vi "Main Tclk.vi"() -> ()   [LabVIEW 2018] (continued)
                n634 = call <vilib>:"Draw Rectangle.vi"("picture"=picture data[5B], "rect"=T46 {"left"=0, "top"=0, "right"=0, "bottom"=0}) -> ("new picture"=w2827:picture)  [unwired: 7 in]
                n635 = Unbundle By Name(w2823) -> ("Primary X index"=w2824:u8[][], "Primary Y index"=w2825:u8[][])
                n636 = case shown="0, Default" w2834 {
                  tunnel: w2829 -> [w2838 w2842]
                  tunnel: [w2837 w2841] -> w2828
                  tunnel: w2827 -> [w2836 w2840]
                  tunnel: [w2835 w2839] -> w2826
                  frame 0, Default {
                    n637 = Unbundle By Name(w2838) -> ("A Img Focus Index array"=w2837:dbl[][])
                    n638 = control-ref of="Detector A"() -> (w2835:refnum<vi>)
                    n639 = property on="Detector B" class="IntGraph (strict)"("PlotImages.Front"=w2836) -> ()  [unwired: 2 in, 2 out]
                  }
                  frame 1 {
                    n640 = Unbundle By Name(w2842) -> ("B Img Focus Index array"=w2841:dbl[][])
                    n641 = control-ref of="Detector B"() -> (w2839:refnum<vi>)
                    n642 = property on="Detector A" class="IntGraph (strict)"("PlotImages.Front"=w2840) -> ()  [unwired: 2 in, 2 out]
                  }
                }
                n643 = Index Array(array=w2818) -> (element #1=w2817:u8, element #2=w2816:u8)  [unwired: 2 in]
                n644 = Index Array(array=w2824, index (row)=w2817, index (col)=w2816) -> (element=w2822:u8)
                n645 = Index Array(array=w2825, index (row)=w2817, index (col)=w2816) -> (element=w2821:u8)
                n646 = call "Display array on Figure.vi"("Y resolution"=w2819, "X resolution"=w2820, "format string"="%2.3f", "Image fit to"=w2815, "Primary grid @ green"=TRUE, "Input array"=w2828, "Primary Y"=w2821, "Primary X"=w2822, "Image reference"=w2826) -> ()  [unwired: 3 in]
              }
              frame #1 {
                n647 = local read "SEM Scan Parameters"() -> (w2845:T26)
                n648 = local read "Focus Index Options"() -> (w2844:T28)
                n649 = local read "Tiled Image fit to"() -> (w2843:u8)
                n650 = call <vilib>:"Draw Rectangle.vi"("picture"=picture data[5B], "rect"=T46 {"left"=0, "top"=0, "right"=0, "bottom"=0}) -> ("new picture"=w2847:picture)  [unwired: 7 in]
                n651 = case shown="0, Default" w2850 {
                  tunnel: w2847 -> [w2852 w2854]
                  tunnel: [w2851 w2853] -> w2846
                  frame 0, Default {
                    n652 = control-ref of="Det A"() -> (w2851:refnum<vi>)
                    n653 = property on="Det B" class="IntGraph (strict)"("PlotImages.Front"=w2852) -> ()  [unwired: 2 in, 2 out]
                  }
                  frame 1 {
                    n654 = control-ref of="Det B"() -> (w2853:refnum<vi>)
                    n655 = property on="Det A" class="IntGraph (strict)"("PlotImages.Front"=w2854) -> ()  [unwired: 2 in, 2 out]
                  }
                }
                n656 = call "Display FI locations on tiled image.vi"("Tiled Image fit to"=w2843, "Focus Index Options"=w2844, "SEM Scan Parameters"=w2845, "Image reference"=w2846) -> ()  [unwired: 8 in]
              }
            }
          }
        }
        n657 = case shown="True" w2528 {
          tunnel: w2526 -> [_ w2750]
          frame False {
          }
          frame True {
            "Last good FI" <- w2750
          }
        }
        n658 = shared-variable "My Computer\\Zeiss Library.lvlib\\Image Fit to"("Image fit to") -> ()  [unwired: 1 in, 1 out]
        n659 = case shown="1" "Image fit to" {
          frame 0, Default {
            n660 = stacked-sequence {
              frame #0 {
                w2688 = u8 0 ("Y Scale.Scale Fit")
                w2689 = u8 1 ("X Scale.Scale Fit")
                n661 = property on="Detector A" class="IntGraph (strict)"("XScale.ScaleFit"=w2689) -> ()  [unwired: 2 in, 2 out]
                n662 = property on="Detector A" class="IntGraph (strict)"("YScale.ScaleFit"=w2688) -> ()  [unwired: 2 in, 2 out]
                n663 = property on="Detector B" class="IntGraph (strict)"("XScale.ScaleFit"=w2689) -> ()  [unwired: 2 in, 2 out]
                n664 = property on="Detector B" class="IntGraph (strict)"("YScale.ScaleFit"=w2688) -> ()  [unwired: 2 in, 2 out]
              }
              frame #1 {
                n665 = property on="Detector A" class="IntGraph (strict)"() -> ("XScale.Maximum"=w2691:dbl)  [unwired: 2 in, 2 out]
                n666 = property on="Detector B" class="IntGraph (strict)"() -> ("XScale.Maximum"=w2690:dbl)  [unwired: 2 in, 2 out]
                n667 = property on="Detector A" class="IntGraph (strict)"("YScale.Maximum"=w2691) -> ()  [unwired: 2 in, 2 out]
                n668 = property on="Detector B" class="IntGraph (strict)"("YScale.Maximum"=w2690) -> ()  [unwired: 2 in, 2 out]
              }
            }
          }
          frame 1 {
            n669 = stacked-sequence {
              frame #0 {
                w2692 = u8 1 ("Y Scale.Scale Fit")
                w2693 = u8 0 ("X Scale.Scale Fit")
                n670 = property on="Detector A" class="IntGraph (strict)"("XScale.ScaleFit"=w2693) -> ()  [unwired: 2 in, 2 out]
                n671 = property on="Detector A" class="IntGraph (strict)"("YScale.ScaleFit"=w2692) -> ()  [unwired: 2 in, 2 out]
                n672 = property on="Detector B" class="IntGraph (strict)"("XScale.ScaleFit"=w2693) -> ()  [unwired: 2 in, 2 out]
                n673 = property on="Detector B" class="IntGraph (strict)"("YScale.ScaleFit"=w2692) -> ()  [unwired: 2 in, 2 out]
              }
              frame #1 {
                n674 = property on="Detector A" class="IntGraph (strict)"() -> ("YScale.Maximum"=w2695:dbl)  [unwired: 2 in, 2 out]
                n675 = property on="Detector B" class="IntGraph (strict)"() -> ("YScale.Maximum"=w2694:dbl)  [unwired: 2 in, 2 out]
                n676 = property on="Detector A" class="IntGraph (strict)"("XScale.Maximum"=w2695) -> ()  [unwired: 2 in, 2 out]
                n677 = property on="Detector B" class="IntGraph (strict)"("XScale.Maximum"=w2694) -> ()  [unwired: 2 in, 2 out]
              }
            }
          }
        }
        n678 = local read "Mid Mag SEM"() -> (w2440:T29)
        n679 = Unbundle By Name(w2440) -> ("Mid mag scan"=w2550:bool, "Show MM box"=w2551:bool)
        n680 = local read "Image Tabs"() -> (w2501:T37)
        n681 = And(x=w2548, y=w2550) -> (x .and. y?=w2549:bool)
        n682 = case shown="\"Imaging Quality\"" w2501 {
          frame "All" {
            w2729 = FALSE ("Visible")
            n683 = property on="Image fit to" class="Ring (strict)"("Visible"=w2729) -> ()  [unwired: 2 in, 2 out]
            n684 = property on="Milling Z realtime (V)" class="DigNum (strict)"("Visible"=w2729) -> ()  [unwired: 2 in, 2 out]
          }
          frame "Detector A", Default {
            n685 = property on="Image fit to" class="Ring (strict)"("Visible"=TRUE) -> ()  [unwired: 2 in, 2 out]
            n686 = property on="Milling Z realtime (V)" class="DigNum (strict)"("Visible"=FALSE) -> ()  [unwired: 2 in, 2 out]
          }
          frame "Detector B" {
            n687 = property on="Image fit to" class="Ring (strict)"("Visible"=TRUE) -> ()  [unwired: 2 in, 2 out]
            n688 = property on="Milling Z realtime (V)" class="DigNum (strict)"("Visible"=FALSE) -> ()  [unwired: 2 in, 2 out]
          }
          frame "Detector A Low Mag" {
            w2734 = FALSE ("Visible")
            n689 = property on="Image fit to" class="Ring (strict)"("Visible"=w2734) -> ()  [unwired: 2 in, 2 out]
            n690 = property on="Milling Z realtime (V)" class="DigNum (strict)"("Visible"=w2734) -> ()  [unwired: 2 in, 2 out]
          }
          frame "Detector B Low Mag" {
            w2735 = FALSE ("Visible")
            n691 = property on="Image fit to" class="Ring (strict)"("Visible"=w2735) -> ()  [unwired: 2 in, 2 out]
            n692 = property on="Milling Z realtime (V)" class="DigNum (strict)"("Visible"=w2735) -> ()  [unwired: 2 in, 2 out]
          }
          frame "FIB" {
            n693 = property on="Image fit to" class="Ring (strict)"("Visible"=FALSE) -> ()  [unwired: 2 in, 2 out]
            n694 = property on="Milling Z realtime (V)" class="DigNum (strict)"("Visible"=TRUE) -> ()  [unwired: 2 in, 2 out]
          }
          frame "FIB Milling Offset after Pause" {
            w2738 = FALSE ("Visible")
            n695 = property on="Image fit to" class="Ring (strict)"("Visible"=w2738) -> ()  [unwired: 2 in, 2 out]
            n696 = property on="Milling Z realtime (V)" class="DigNum (strict)"("Visible"=w2738) -> ()  [unwired: 2 in, 2 out]
          }
          frame "Auto Focus / Stig / Align" {
            w2739 = FALSE ("Visible")
            n697 = property on="Image fit to" class="Ring (strict)"("Visible"=w2739) -> ()  [unwired: 2 in, 2 out]
            n698 = property on="Milling Z realtime (V)" class="DigNum (strict)"("Visible"=w2739) -> ()  [unwired: 2 in, 2 out]
          }
          frame "Imaging Quality" {
            w2740 = FALSE ("Visible")
            n699 = property on="Image fit to" class="Ring (strict)"("Visible"=w2740) -> ()  [unwired: 2 in, 2 out]
            n700 = property on="Milling Z realtime (V)" class="DigNum (strict)"("Visible"=w2740) -> ()  [unwired: 2 in, 2 out]
          }
          frame "Temp. and Currents" {
            w2741 = FALSE ("Visible")
            n701 = property on="Image fit to" class="Ring (strict)"("Visible"=w2741) -> ()  [unwired: 2 in, 2 out]
            n702 = property on="Milling Z realtime (V)" class="DigNum (strict)"("Visible"=w2741) -> ()  [unwired: 2 in, 2 out]
          }
          frame "FIB HV Data" {
            w2742 = FALSE ("Visible")
            n703 = property on="Image fit to" class="Ring (strict)"("Visible"=w2742) -> ()  [unwired: 2 in, 2 out]
            n704 = property on="Milling Z realtime (V)" class="DigNum (strict)"("Visible"=w2742) -> ()  [unwired: 2 in, 2 out]
          }
          frame "Logging: Realtime Graphs" {
            n705 = property on="Image fit to" class="Ring (strict)"("Visible"=FALSE) -> ()  [unwired: 2 in, 2 out]
            n706 = property on="Milling Z realtime (V)" class="DigNum (strict)"("Visible"=TRUE) -> ()  [unwired: 2 in, 2 out]
          }
        }
        n707 = case shown="False" w2549 {
          tunnel: [T44."Disabled and Grayed Out" ("Disabled") T44."Enabled" ("Disabled")] -> w2552
          tunnel: w2440 -> [w2768 _]
          frame False {
            n708 = Bundle By Name(cluster=w2768, "Show MM box"=FALSE ("Show HM box")) -> (w2767:T29)
            n709 = local write "Mid Mag SEM"(w2767) -> ()
          }
          frame True {
          }
        }
        n710 = local read "Load recipe"() -> (w2470:bool)
        n711 = property on="Show MM box" class="Bool (strict)"("DisabledEnum"=w2552) -> ()  [unwired: 2 in, 2 out]
        n712 = case shown="False" w2470 {
          frame False {
            n713 = local read "X shift (nm/image)"() -> (w2726:sgl)
            n714 = local read "Y shift (nm/image)"() -> (w2727:sgl)
            n715 = local read "SEM Scan Parameters"() -> (w2718:T26)
            n716 = local read "Detector Information"() -> (w2699:T8)
            n717 = local read "SEM Options"() -> (w2717:T27)
            n718 = local read "Focus Index Options"() -> (w2698:T28)
            n719 = local read "Image fit to"() -> (w2703:u8)
            n720 = local read "File Information"() -> (w2716:T31)
            n721 = local read "Low Mag SEM"() -> (w2715:T30)
            n722 = local read "Mid Mag SEM"() -> (w2709:T29)
            n723 = local read "FIB-SEM Angle"() -> (w2714:dbl)
            n724 = local read "Milling para"() -> (w2713:T35)
            n725 = local read "FI Detector"() -> (w2719:u16)
            n726 = local read "Auto Optimzation"() -> (w2720:bool)
            n727 = local read "Images per Auto Optimization"() -> (w2721:u16)
            n728 = local read "AF Range (nm)"() -> (w2722:sgl)
            n729 = local read "AF Steps"() -> (w2723:u8)
            n730 = local read "AS Range (%)"() -> (w2724:sgl)
            n731 = local read "AS Steps"() -> (w2725:u8)
            n732 = local read "AA Range (%)"() -> (w2705:sgl)
            n733 = local read "AA Steps"() -> (w2704:u8)
            n734 = local read "FIB Y zoom pixel (nm)"() -> (w2712:dbl)
            n735 = local read "Mail server"() -> (w2711:string)
            n736 = local read "Email Alert Recipients"() -> (w2710:string[])
            n737 = local read "Alert Settings"() -> (w2708:T36)
            n738 = local read "Reheat Parameters"() -> (w2702:T1)
            n739 = local read "Start FIB HV DataLog"() -> (w2701:bool)
            n740 = local read "Interval (s)"() -> (w2700:u16)
            n741 = Bundle By Name(cluster="Recipe input", "SEM Scan Parameters"=w2718, "Detector Information"=w2699, "SEM Options"=w2717, "Focus Index Options"=w2698, "Image fit to"=w2703, "File Information"=w2716, "Low mag SEM"=w2715, "Mid Mag SEM"=w2709, "FIB-SEM Angle"=w2714, "Milling para"=w2713, "FI Detector"=w2719, "Auto Optimzation"=w2720, "Images per Auto Optimization"=w2721, "AF Range (nm)"=w2722, "AF Steps"=w2723, "AS Range (%)"=w2724, "AS Steps"=w2725, "AA Range (%)"=w2705, "AA Steps"=w2704, "X shift (nm/frame)"=w2726, "Y shift (nm/frame)"=w2727, "FIB Y zoom pixel (nm)"=w2712, "Mail server"=w2711, "Email Alert Recipents"=w2710, "Alert Settings"=w2708, "Reheat Parameters"=w2702, "Start FIB HV DataLog"=w2701, "Interval (s)"=w2700) -> (w2707:T7)
            n742 = To Variant(anything=w2707) -> (Variant=w2706:variant)
            n743 = shared-variable ".\\Zeiss Library.lvlib\\Recipe input"(w2706) -> ()  [unwired: 1 in, 1 out]
            n744 = local write "Recipe input"(w2707) -> ()
          }
          frame True {
          }
        }
        n745 = case shown="True" w2551 {
          tunnel: w2554 -> [w2772 w2778]
          tunnel: w2553 -> [w2771 w2776]
          tunnel: [w2772 w2777] -> w2542
          tunnel: [w2771 w2775] -> w2541
          frame False {
          }
          frame True {
            w2789 = T46 {"left"=0, "top"=0, "right"=0, "bottom"=0} ("rect")
            n746 = property on="Det A LM" class="IntGraph (strict)"() -> ("Width"=w2802:u32, "Height"=w2806:u32)  [unwired: 2 in, 2 out]
            n747 = local read "Low Mag SEM"() -> (w2780:T30)
            n748 = local read "Mid Mag SEM"() -> (w2803:T29)
            n749 = property on="Detector A Low Mag" class="IntGraph (strict)"() -> ("Width"=w2784:u32, "Height"=w2783:u32)  [unwired: 2 in, 2 out]
            n750 = Unbundle By Name(w2780) -> ("Low mag scan FOV (micron)"=w2779:dbl)
            n751 = Unbundle By Name(w2803) -> ("X center (um)"=w2807:dbl, "Y center (um)"=w2808:dbl, "X size (um)"=w2774:sgl, "Y size (um)"=w2773:sgl)
            n752 = expression code="x/2"(w2779) -> (w2809:dbl)
            n753 = Divide(x=w2807, y=w2809) -> (x/y=w2786:dbl)
            n754 = Divide(x=w2808, y=w2809) -> (x/y=w2782:dbl)
            n755 = Divide(x=w2774, y=w2809) -> (x/y=w2785:dbl)
            n756 = Divide(x=w2773, y=w2809) -> (x/y=w2781:dbl)
            n757 = call "CenterSize to StartEnd or Rect-4C.vi"("Resolution"=w2802, "Size"=w2785, "Center"=w2786) -> ("Rect-4C"=w2805:cluster{"left":i16, "right":i16})  [unwired: 2 in, 2 out]
            n758 = call "CenterSize to StartEnd or Rect-4C.vi"("Resolution"=w2806, "Size"=w2781, "Center"=w2782) -> ("Rect-4C"=w2804:cluster{"left":i16, "right":i16})  [unwired: 2 in, 2 out]
            n759 = call "CenterSize to StartEnd or Rect-4C.vi"("Resolution"=w2784, "Size"=w2785, "Center"=w2786) -> ("Rect-4C"=w2790:cluster{"left":i16, "right":i16})  [unwired: 2 in, 2 out]
            n760 = call "CenterSize to StartEnd or Rect-4C.vi"("Resolution"=w2783, "Size"=w2781, "Center"=w2782) -> ("Rect-4C"=w2791:cluster{"left":i16, "right":i16})  [unwired: 2 in, 2 out]
            n761 = Unbundle(w2805) -> ("left"=w2800:i16, "right"=w2799:i16)
            n762 = Unbundle(w2804) -> ("left"=w2798:i16, "right"=w2797:i16)
            n763 = Unbundle(w2790) -> ("left"=w2792:i16, "right"=w2793:i16)
            n764 = Unbundle(w2791) -> ("left"=w2794:i16, "right"=w2795:i16)
            n765 = Bundle By Name(cluster=w2789, "left"=w2800, "right"=w2799, "top"=w2798, "bottom"=w2797) -> (w2796:T46)
            n766 = Bundle By Name(cluster=w2789, "left"=w2792, "right"=w2793, "top"=w2794, "bottom"=w2795) -> (w2787:T46)
            n767 = call <vilib>:"Draw Rectangle.vi"("picture"=w2778, "rect"=w2796, "color(black)"=u32 3381759) -> ("new picture"=w2777:picture)  [unwired: 6 in]
            n768 = call <vilib>:"Draw Rectangle.vi"("picture"=w2776, "rect"=w2787, "color(black)"=u32 3381759) -> ("new picture"=w2775:picture)  [unwired: 6 in]
          }
        }
        n769 = call <vilib>:"Draw Rectangle.vi"("picture"=picture data[5B], "rect"=T46 {"left"=0, "top"=0, "right"=0, "bottom"=0}) -> ("new picture"=w2538:picture)  [unwired: 7 in]
        n770 = local read "SEM Options"() -> (w2555:T27)
        n771 = local read "Hardware Configuration"() -> (w2450:T25)
        n772 = Unbundle By Name(w2450) -> ("Brightness A"=w2449:dbl, "Contrast A"=w2448:dbl, "Detector B name"=w2447:string, "Brightness B"=w2446:dbl, "Contrast B"=w2445:dbl)
        n773 = local read "Machine Type"() -> (w2414:u8)
        n774 = local read "SEM Scan Parameters"() -> (w2422:T26)
        n775 = local read "SEM scan time"() -> (w2425:dbl)
        n776 = local read "Milling time (s)"() -> (w2418:sgl)
        n777 = local read "Focus Index Options"() -> (w2403:T28)
        n778 = Unbundle By Name(w2555) -> ("Detector A"=w2557:bool, "Detector B"=w2558:bool)
        n779 = Bundle By Name(cluster="Detector Information", "Brightness A"=w2449, "Contrast A"=w2448, "Detector B name"=w2447, "Brightness B"=w2446, "Contrast B"=w2445) -> (w2443:T8)
        n780 = case shown="2" w2414 {
          tunnel: [u8 3 ("x*y") u8 3 ("x*y") u8 2 ("x*y")] -> w2413
          frame 0, Default {
          }
          frame 1 {
          }
          frame 2 {
          }
        }
        n781 = Unbundle By Name(w2422) -> ("X tiles"=w2420:u8, "Y tiles"=w2423:u8, "Frames"=w2426:u8)
        n782 = Build Array(w2557, w2558) -> (w2556:bool[])
        n783 = Unbundle By Name(w2403) -> ("Focus Index primary grid center"=w2408:bool, "X Grids"=w2407:u8[][], "Primary X index"=w2406:u8[][], "Y Grids"=w2405:u8[][], "Primary Y index"=w2404:u8[][])
        n784 = Boolean Array To Number(Boolean array=w2556) -> (number=w2540:u32)
        n785 = Multiply(x=w2420, y=w2423) -> (x*y=w2417:u8)
        n786 = Multiply(x=w2426, y=w2425) -> (x*y=w2424:dbl)
        n787 = Decrement(x=w2417) -> (x-1=w2416:u8)
        n788 = local write "Detector Information"(w2443) -> ()
        n789 = Multiply(x=w2413, y=w2416) -> (x*y=w2415:u8)
        n790 = case shown="1, Default" w2540 {
          tunnel: w2542 -> [w2760 w2763 w2765]
          tunnel: w2541 -> [w2759 w2762 w2764]
          tunnel: [w2758 w2763 w2765] -> w2543
          tunnel: [w2760 w2761 w2765] -> w2544
          tunnel: [w2759 w2761 w2764] -> w2545
          tunnel: [w2758 w2762 w2764] -> w2546
          tunnel: w2538 -> [w2758 w2761 _]
          frame 1, Default {
          }
          frame 2 {
          }
          frame 3 {
          }
        }
        n791 = local read "Overhead (s)"() -> (w2419:sgl)
        n792 = property on="Det A LM" class="IntGraph (strict)"("PlotImages.Front"=w2544) -> ()  [unwired: 2 in, 2 out]
        n793 = property on="Det B LM" class="IntGraph (strict)"("PlotImages.Front"=w2543) -> ()  [unwired: 2 in, 2 out]
        n794 = property on="Detector A Low Mag" class="IntGraph (strict)"("PlotImages.Front"=w2545) -> ()  [unwired: 2 in, 2 out]
        n795 = property on="Detector B Low Mag" class="IntGraph (strict)"("PlotImages.Front"=w2546) -> ()  [unwired: 2 in, 2 out]
        n796 = case shown="False" w2408 {
          tunnel: w2407 -> [w2642 w2663]
          tunnel: w2406 -> [w2641 _]
          tunnel: w2405 -> [w2640 w2662]
          tunnel: w2404 -> [w2639 _]
          tunnel: w2403 -> [w2638 w2661]
          frame False {
            n797 = for {
              tunnel: w2642 -> [w2653] mode=indexing
              tunnel: w2641 -> [w2652] mode=indexing
              tunnel: [w2651] -> w2646 mode=indexing
              tunnel: w2640 -> [w2650] mode=indexing
              tunnel: w2639 -> [w2649] mode=indexing
              tunnel: [w2648] -> w2645 mode=indexing
              tunnel: u8 1 ("x") -> [w2647]
              n798 = for {
                tunnel: w2653 -> [w2660] mode=indexing
                tunnel: w2652 -> [w2659] mode=indexing
                tunnel: [w2658] -> w2651 mode=indexing
                tunnel: w2650 -> [w2657] mode=indexing
                tunnel: w2649 -> [w2656] mode=indexing
                tunnel: [w2655] -> w2648 mode=indexing
                tunnel: w2647 -> [w2654]
                n799 = In Range and Coerce(upper limit=w2660, x=w2659, lower limit=w2654) -> (coerced(x)=w2658:u8)  [unwired: 1 out]
                n800 = In Range and Coerce(upper limit=w2657, x=w2656, lower limit=w2654) -> (coerced(x)=w2655:u8)  [unwired: 1 out]
              }
            }
            n801 = Bundle By Name(cluster=w2638, "Primary X index"=w2646, "Primary Y index"=w2645) -> (w2644:T28)
            n802 = local write "Focus Index Options"(w2644) -> ()
          }
          frame True {
            n803 = for {
              tunnel: w2663 -> [w2674] mode=indexing
              tunnel: w2662 -> [w2673] mode=indexing
              tunnel: [w2672] -> w2667 mode=indexing
              tunnel: [w2671] -> w2666 mode=indexing
              tunnel: [w2670] -> w2665 mode=indexing
              tunnel: [w2669] -> w2664 mode=indexing
              n804 = for {
                tunnel: w2674 -> [w2680] mode=indexing
                tunnel: w2673 -> [w2679] mode=indexing
                tunnel: [w2678] -> w2672 mode=indexing
                tunnel: [w2677] -> w2671 mode=indexing
                tunnel: [w2676] -> w2670 mode=indexing
                tunnel: [w2675] -> w2669 mode=indexing
                n805 = To Single Precision Float(number=w2680) -> (single precision float=w2683:sgl)
                n806 = To Single Precision Float(number=w2679) -> (single precision float=w2682:sgl)
                n807 = expression code="x/2"(w2683) -> (w2684:sgl)
                n808 = expression code="x/2"(w2682) -> (w2681:sgl)
                n809 = Round Toward +Infinity(x=w2684) -> (ceil(x): smallest int >= x=w2677:sgl)
                n810 = Round Toward +Infinity(x=w2681) -> (ceil(x): smallest int >= x=w2675:sgl)
                n811 = expression code="x*2-1"(w2677) -> (w2678:sgl)
                n812 = expression code="x*2-1"(w2675) -> (w2676:sgl)
              }
            }
            n813 = Bundle By Name(cluster=w2661, "X Grids"=w2667, "Primary X index"=w2666, "Y Grids"=w2665, "Primary Y index"=w2664) -> (w2668:T28)
            n814 = local write "Focus Index Options"(w2668) -> ()
          }
        }
        n815 = local read "SEM Options"() -> (w2525:T27)
        n816 = local read "SEM Parameters"() -> (w2630:T13)
        n817 = local read "Detector Information"() -> (w2629:T8)
        n818 = Compound Arithmetic op=ADD(w2419, w2415, w2424, w2418) -> (→"Est. cycle time (s)":dbl)
        n819 = shared-variable "My Computer\\Zeiss Library.lvlib\\Milling Post-pause Lines"() -> (→"Rect Milling Post-pause Lines":u16)  [unwired: 1 in, 1 out]
        n820 = shared-variable ".\\Zeiss Library.lvlib\\Realtime Imaging Info"() -> (w2596:variant)  [unwired: 1 in, 1 out]
        n821 = shared-variable ".\\Zeiss Library.lvlib\\Milling Progress"() -> (w2595:u8[])  [unwired: 1 in, 1 out]
        n822 = local read "SEM Status"() -> (w2474:T12)
        n823 = Unbundle By Name(w2525) -> ("8-bit"=w2409:bool, "Inverse A"=w2615:bool, "Inverse B"=w2599:bool)
        n824 = Unbundle By Name(w2630) -> ("Detector A"=w2635:string)
        n825 = Unbundle By Name(w2629) -> ("Detector B name"=w2636:string)
        n826 = Unbundle By Name(w2474) -> ("Y tile"=w2473:u8, "X tile"=w2472:u8)
        n827 = property on="DetA e- Scaling" class="DigNum (strict)"("Visible"=w2409) -> ()  [unwired: 2 in, 2 out]
        n828 = Select(t=u32[] [16448250, 16711422, 16645629, 16579836, 16514043, 16448250, 16382457, 16316664, 16250871, 16185078, 16119285, 16053492, 15987699, 15921906, 15856113, 15790320, 15724527, 15658734, 15592941, 15527148, 15461355, 15395562, 15329769, 15263976, 15198183, 15132390, 15066597, 15000804, 14935011, 14869218, 14803425, 14737632, 14671839, 14606046, 14540253, 14474460, 14408667, 14342874, 14277081, 14211288, 14145495, 14079702, 14013909, 13948116, 13882323, 13816530, 13750737, 13684944, 13619151, 13553358, 13487565, 13421772, 13355979, 13290186, 13224393, 13158600, 13092807, 13027014, 12961221, 12895428, 12829635, 12763842, 12698049, 12632256, 12566463, 12500670, 12434877, 12369084, 12303291, 12237498, 12171705, 12105912, 12040119, 11974326, 11908533, 11842740, 11776947, 11711154, 11645361, 11579568, 11513775, 11447982, 11382189, 11316396, 11250603, 11184810, 11119017, 11053224, 10987431, 10921638, 10855845, 10790052, 10724259, 10658466, 10592673, 10526880, 10461087, 10395294, 10329501, 10263708, 10197915, 10132122, 10066329, 10000536, 9934743, 9868950, 9803157, 9737364, 9671571, 9605778, 9539985, 9474192, 9408399, 9342606, 9276813, 9211020, 9145227, 9079434, 9013641, 8947848, 8882055, 8816262, 8750469, 8684676, 8618883, 8553090, 8487297, 8421504, 8355711, 8289918, 8224125, 8158332, 8092539, 8026746, 7960953, 7895160, 7829367, 7763574, 7697781, 7631988, 7566195, 7500402, 7434609, 7368816, 7303023, 7237230, 7171437, 7105644, 7039851, 6974058, 6908265, 6842472, 6776679, 6710886, 6645093, 6579300, 6513507, 6447714, 6381921, 6316128, 6250335, 6184542, 6118749, 6052956, 5987163, 5921370, 5855577, 5789784, 5723991, 5658198, 5592405, 5526612, 5460819, 5395026, 5329233, 5263440, 5197647, 5131854, 5066061, 5000268, 4934475, 4868682, 4802889, 4737096, 4671303, 4605510, 4539717, 4473924, 4408131, 4342338, 4276545, 4210752, 4144959, 4079166, 4013373, 3947580, 3881787, 3815994, 3750201, 3684408, 3618615, 3552822, 3487029, 3421236, 3355443, 3289650, 3223857, 3158064, 3092271, 3026478, 2960685, 2894892, 2829099, 2763306, 2697513, 2631720, 2565927, 2500134, 2434341, 2368548, 2302755, 2236962, 2171169, 2105376, 2039583, 1973790, 1907997, 1842204, 1776411, 1710618, 1644825, 1579032, 1513239, 1447446, 1381653, 1315860, 1250067, 1184274, 1118481, 1052688, 986895, 921102, 855309, 789516, 723723, 657930, 592137, 526344, 460551, 394758, 328965, 263172, 197379, 131586, 65793, 16777222] ("256 gray scale inverse"), s=w2615, f=u32[] [16777222, 65793, 131586, 197379, 263172, 328965, 394758, 460551, 526344, 592137, 657930, 723723, 789516, 855309, 921102, 986895, 1052688, 1118481, 1184274, 1250067, 1315860, 1381653, 1447446, 1513239, 1579032, 1644825, 1710618, 1776411, 1842204, 1907997, 1973790, 2039583, 2105376, 2171169, 2236962, 2302755, 2368548, 2434341, 2500134, 2565927, 2631720, 2697513, 2763306, 2829099, 2894892, 2960685, 3026478, 3092271, 3158064, 3223857, 3289650, 3355443, 3421236, 3487029, 3552822, 3618615, 3684408, 3750201, 3815994, 3881787, 3947580, 4013373, 4079166, 4144959, 4210752, 4276545, 4342338, 4408131, 4473924, 4539717, 4605510, 4671303, 4737096, 4802889, 4868682, 4934475, 5000268, 5066061, 5131854, 5197647, 5263440, 5329233, 5395026, 5460819, 5526612, 5592405, 5658198, 5723991, 5789784, 5855577, 5921370, 5987163, 6052956, 6118749, 6184542, 6250335, 6316128, 6381921, 6447714, 6513507, 6579300, 6645093, 6710886, 6776679, 6842472, 6908265, 6974058, 7039851, 7105644, 7171437, 7237230, 7303023, 7368816, 7434609, 7500402, 7566195, 7631988, 7697781, 7763574, 7829367, 7895160, 7960953, 8026746, 8092539, 8158332, 8224125, 8289918, 8355711, 8421504, 8487297, 8553090, 8618883, 8684676, 8750469, 8816262, 8882055, 8947848, 9013641, 9079434, 9145227, 9211020, 9276813, 9342606, 9408399, 9474192, 9539985, 9605778, 9671571, 9737364, 9803157, 9868950, 9934743, 10000536, 10066329, 10132122, 10197915, 10263708, 10329501, 10395294, 10461087, 10526880, 10592673, 10658466, 10724259, 10790052, 10855845, 10921638, 10987431, 11053224, 11119017, 11184810, 11250603, 11316396, 11382189, 11447982, 11513775, 11579568, 11645361, 11711154, 11776947, 11842740, 11908533, 11974326, 12040119, 12105912, 12171705, 12237498, 12303291, 12369084, 12434877, 12500670, 12566463, 12632256, 12698049, 12763842, 12829635, 12895428, 12961221, 13027014, 13092807, 13158600, 13224393, 13290186, 13355979, 13421772, 13487565, 13553358, 13619151, 13684944, 13750737, 13816530, 13882323, 13948116, 14013909, 14079702, 14145495, 14211288, 14277081, 14342874, 14408667, 14474460, 14540253, 14606046, 14671839, 14737632, 14803425, 14869218, 14935011, 15000804, 15066597, 15132390, 15198183, 15263976, 15329769, 15395562, 15461355, 15527148, 15592941, 15658734, 15724527, 15790320, 15856113, 15921906, 15987699, 16053492, 16119285, 16185078, 16250871, 16316664, 16382457, 16448250, 16514043, 16579836, 16645629, 16711422, 16448250] ("256 gray scale")) -> (s? t:f=w2601:u32[])
        n829 = Variant To Data(Variant=w2596) -> (data=→"FIB Status":T20)  [unwired: 2 in, 1 out]
        n830 = Index Array(array=w2595) -> (element #1=→"Line progress":u8, element #2=→"Total progress":u8)  [unwired: 2 in]
        n831 = Build Array(w2473, w2472) -> (w2471:u8[])
        n832 = property on="Detector A" class="IntGraph (strict)"("Color Table"=w2601, "Caption.Text"=w2635) -> ()  [unwired: 2 in, 2 out]
        n833 = Select(t=u32[] [16448250, 16711422, 16645629, 16579836, 16514043, 16448250, 16382457, 16316664, 16250871, 16185078, 16119285, 16053492, 15987699, 15921906, 15856113, 15790320, 15724527, 15658734, 15592941, 15527148, 15461355, 15395562, 15329769, 15263976, 15198183, 15132390, 15066597, 15000804, 14935011, 14869218, 14803425, 14737632, 14671839, 14606046, 14540253, 14474460, 14408667, 14342874, 14277081, 14211288, 14145495, 14079702, 14013909, 13948116, 13882323, 13816530, 13750737, 13684944, 13619151, 13553358, 13487565, 13421772, 13355979, 13290186, 13224393, 13158600, 13092807, 13027014, 12961221, 12895428, 12829635, 12763842, 12698049, 12632256, 12566463, 12500670, 12434877, 12369084, 12303291, 12237498, 12171705, 12105912, 12040119, 11974326, 11908533, 11842740, 11776947, 11711154, 11645361, 11579568, 11513775, 11447982, 11382189, 11316396, 11250603, 11184810, 11119017, 11053224, 10987431, 10921638, 10855845, 10790052, 10724259, 10658466, 10592673, 10526880, 10461087, 10395294, 10329501, 10263708, 10197915, 10132122, 10066329, 10000536, 9934743, 9868950, 9803157, 9737364, 9671571, 9605778, 9539985, 9474192, 9408399, 9342606, 9276813, 9211020, 9145227, 9079434, 9013641, 8947848, 8882055, 8816262, 8750469, 8684676, 8618883, 8553090, 8487297, 8421504, 8355711, 8289918, 8224125, 8158332, 8092539, 8026746, 7960953, 7895160, 7829367, 7763574, 7697781, 7631988, 7566195, 7500402, 7434609, 7368816, 7303023, 7237230, 7171437, 7105644, 7039851, 6974058, 6908265, 6842472, 6776679, 6710886, 6645093, 6579300, 6513507, 6447714, 6381921, 6316128, 6250335, 6184542, 6118749, 6052956, 5987163, 5921370, 5855577, 5789784, 5723991, 5658198, 5592405, 5526612, 5460819, 5395026, 5329233, 5263440, 5197647, 5131854, 5066061, 5000268, 4934475, 4868682, 4802889, 4737096, 4671303, 4605510, 4539717, 4473924, 4408131, 4342338, 4276545, 4210752, 4144959, 4079166, 4013373, 3947580, 3881787, 3815994, 3750201, 3684408, 3618615, 3552822, 3487029, 3421236, 3355443, 3289650, 3223857, 3158064, 3092271, 3026478, 2960685, 2894892, 2829099, 2763306, 2697513, 2631720, 2565927, 2500134, 2434341, 2368548, 2302755, 2236962, 2171169, 2105376, 2039583, 1973790, 1907997, 1842204, 1776411, 1710618, 1644825, 1579032, 1513239, 1447446, 1381653, 1315860, 1250067, 1184274, 1118481, 1052688, 986895, 921102, 855309, 789516, 723723, 657930, 592137, 526344, 460551, 394758, 328965, 263172, 197379, 131586, 65793, 16777222] ("256 gray scale inverse"), s=w2599, f=u32[] [16777222, 65793, 131586, 197379, 263172, 328965, 394758, 460551, 526344, 592137, 657930, 723723, 789516, 855309, 921102, 986895, 1052688, 1118481, 1184274, 1250067, 1315860, 1381653, 1447446, 1513239, 1579032, 1644825, 1710618, 1776411, 1842204, 1907997, 1973790, 2039583, 2105376, 2171169, 2236962, 2302755, 2368548, 2434341, 2500134, 2565927, 2631720, 2697513, 2763306, 2829099, 2894892, 2960685, 3026478, 3092271, 3158064, 3223857, 3289650, 3355443, 3421236, 3487029, 3552822, 3618615, 3684408, 3750201, 3815994, 3881787, 3947580, 4013373, 4079166, 4144959, 4210752, 4276545, 4342338, 4408131, 4473924, 4539717, 4605510, 4671303, 4737096, 4802889, 4868682, 4934475, 5000268, 5066061, 5131854, 5197647, 5263440, 5329233, 5395026, 5460819, 5526612, 5592405, 5658198, 5723991, 5789784, 5855577, 5921370, 5987163, 6052956, 6118749, 6184542, 6250335, 6316128, 6381921, 6447714, 6513507, 6579300, 6645093, 6710886, 6776679, 6842472, 6908265, 6974058, 7039851, 7105644, 7171437, 7237230, 7303023, 7368816, 7434609, 7500402, 7566195, 7631988, 7697781, 7763574, 7829367, 7895160, 7960953, 8026746, 8092539, 8158332, 8224125, 8289918, 8355711, 8421504, 8487297, 8553090, 8618883, 8684676, 8750469, 8816262, 8882055, 8947848, 9013641, 9079434, 9145227, 9211020, 9276813, 9342606, 9408399, 9474192, 9539985, 9605778, 9671571, 9737364, 9803157, 9868950, 9934743, 10000536, 10066329, 10132122, 10197915, 10263708, 10329501, 10395294, 10461087, 10526880, 10592673, 10658466, 10724259, 10790052, 10855845, 10921638, 10987431, 11053224, 11119017, 11184810, 11250603, 11316396, 11382189, 11447982, 11513775, 11579568, 11645361, 11711154, 11776947, 11842740, 11908533, 11974326, 12040119, 12105912, 12171705, 12237498, 12303291, 12369084, 12434877, 12500670, 12566463, 12632256, 12698049, 12763842, 12829635, 12895428, 12961221, 13027014, 13092807, 13158600, 13224393, 13290186, 13355979, 13421772, 13487565, 13553358, 13619151, 13684944, 13750737, 13816530, 13882323, 13948116, 14013909, 14079702, 14145495, 14211288, 14277081, 14342874, 14408667, 14474460, 14540253, 14606046, 14671839, 14737632, 14803425, 14869218, 14935011, 15000804, 15066597, 15132390, 15198183, 15263976, 15329769, 15395562, 15461355, 15527148, 15592941, 15658734, 15724527, 15790320, 15856113, 15921906, 15987699, 16053492, 16119285, 16185078, 16250871, 16316664, 16382457, 16448250, 16514043, 16579836, 16645629, 16711422, 16448250] ("256 gray scale")) -> (s? t:f=w2600:u32[])
        n834 = property on="DetB e- Scaling" class="DigNum (strict)"("Visible"=w2409) -> ()  [unwired: 2 in, 2 out]
        n835 = property on="Detector B" class="IntGraph (strict)"("Color Table"=w2600, "Caption.Text"=w2636) -> ()  [unwired: 2 in, 2 out]
        n836 = property on="Det A" class="IntGraph (strict)"("Color Table"=w2601) -> ()  [unwired: 2 in, 2 out]
        n837 = property on="Align failed array" class="Arr (strict)"("Index Values"=w2471) -> ()  [unwired: 2 in, 2 out]
        n838 = property on="WD (mm)" class="Arr (strict)"("Index Values"=w2471) -> ()  [unwired: 2 in, 2 out]
        n839 = property on="X stig" class="Arr (strict)"("Index Values"=w2471) -> ()  [unwired: 2 in, 2 out]
        n840 = property on="Y stig" class="Arr (strict)"("Index Values"=w2471) -> ()  [unwired: 2 in, 2 out]
        n841 = property on="X aln" class="Arr (strict)"("Index Values"=w2471) -> ()  [unwired: 2 in, 2 out]
        n842 = property on="Y aln" class="Arr (strict)"("Index Values"=w2471) -> ()  [unwired: 2 in, 2 out]
        n843 = property on="Det B" class="IntGraph (strict)"("Color Table"=w2600) -> ()  [unwired: 2 in, 2 out]
        n844 = property on="Detector A Low Mag" class="IntGraph (strict)"("Color Table"=w2601) -> ()  [unwired: 2 in, 2 out]
        n845 = local read "FIB"() -> (w2411:bool)
        n846 = local read "Mill"() -> (w2410:bool)
        n847 = property on="Detector B Low Mag" class="IntGraph (strict)"("Color Table"=w2600) -> ()  [unwired: 2 in, 2 out]
        n848 = Or(x=w2411, y=w2410) -> (x .or. y?=w2412:bool)
        n849 = shared-variable ".\\Zeiss Library.lvlib\\Milling Z Voltage RT"() -> (w2527:sgl)  [unwired: 1 in, 1 out]
        "Milling Z realtime (V)" <- w2527
        n850 = case shown="True" w2412 {
          tunnel: w2527 -> [_ w2745]
          frame False {
          }
          frame True {
            n851 = control-ref of="FIB Image"() -> (w2749:refnum<vi>)
            n852 = local read "FIB Scan Parameters"() -> (w2747:T32)
            n853 = local read "FIB Options"() -> (w2746:T33)
            n854 = local read "Milling para"() -> (w2748:T35)
            n855 = call "FIB image draw milling.vi"("Milling Z Voltage"=w2745, "Milling para"=w2748, "FIB Options"=w2746, "FIB Scan Parameters"=w2747, "Image reference"=w2749) -> ()  [unwired: 5 in, 2 out]
          }
        }
        n856 = property on="Det A LM" class="IntGraph (strict)"("Color Table"=w2601) -> ()  [unwired: 2 in, 2 out]
        n857 = property on="Det B LM" class="IntGraph (strict)"("Color Table"=w2600) -> ()  [unwired: 2 in, 2 out]
      }
      n858 = while {
        stop <- w717 stop-if-true
        n859 = Wait Until Next ms Multiple(millisecond multiple=u32 100) -> ()  [unwired: 1 out]
        n860 = case shown="True" "Scan x1" {
          frame False {
          }
          frame True {
            n861 = Two Button Dialog(message="Single SEM Scan?") -> (T button?=w720:bool)  [unwired: 2 in]
            n862 = case shown="True" w720 {
              frame False {
                n863 = local write "Scan x1"(FALSE ("Scan")) -> ()
              }
              frame True {
                n864 = stacked-sequence {
                  seq-local: [w728 _ _] -> [_ w739 _]
                  seq-local: [_ w738 _] -> [_ _ w747]
                  seq-local: [_ w737 _] -> [_ _ w746]
                  frame #0 {
                    n865 = local read "SEM HW Config"() -> (w731:T9)
                    n866 = local read "Detector Information"() -> (w730:T8)
                    n867 = local read "SEM Scan Parameters"() -> (w727:T26)
                    n868 = local read "SEM Options"() -> (w726:T27)
                    n869 = local read "Focus Index Options"() -> (w725:T28)
                    n870 = local read "File Information"() -> (w724:T31)
                    n871 = local read "Milling para"() -> (w723:T35)
                    n872 = Bundle By Name(cluster="Tiled scan inputs", "HW Config"=w731, "Det Info"=w730, "SEM Scan Parameters"=w727, "SEM Options"=w726, "Focus Index Options"=w725, "File Information"=w724, "Milling para"=w723) -> (w728:T6)
                  }
                  frame #1 {
                    n873 = call "2D scan tiled.vi"("Tiled scan inputs"=w739) -> ("Image Focus Index Tiled"=w738:T52, "Image Focus Index Array Tiled"=w737:T53, "Single scan outputs"=w742:T54, "8-bit over scale"=w736:bool[])  [unwired: 5 in, 2 out]
                    n874 = Unbundle By Name(w742) -> ("SEM Parameters"=→"SEM Parameters":T13, "Image Focus Index"=→"Image Focus Index":T14)
                    n875 = Index Array(array=w736, index #1=0 ("index"), index #2=1 ("index")) -> (element #1=→"Det A over scale":bool, element #2=→"Det B over scale":bool)
                    "Status message" <- "SEM scanning" ("Status message")
                  }
                  frame #2 {
                    n876 = local read "FI Detector"() -> (w748:u16)
                    n877 = case shown="0, Default" w748 {
                      tunnel: w747 -> [w754 w758 w762 w766]
                      tunnel: [w753 w755 w761 w765] -> w745
                      tunnel: w746 -> [w751 w757 w760 w764]
                      tunnel: [w752 w756 w759 w763] -> w744
                      frame 0, Default {
                        n878 = Unbundle By Name(w754) -> ("A Img Focus Index"=w753:sgl[][])
                        n879 = Unbundle By Name(w751) -> ("A Img Focus Index array"=w752:sgl[][][][])
                      }
                      frame 1 {
                        n880 = Unbundle By Name(w758) -> ("B Img Focus Index"=w755:sgl[][])
                        n881 = Unbundle By Name(w757) -> ("B Img Focus Index array"=w756:sgl[][][][])
                      }
                      frame 2 {
                        n882 = Unbundle By Name(w762) -> ("C Img Focus Index"=w761:sgl[][])
                        n883 = Unbundle By Name(w760) -> ("C Img Focus Index array"=w759:sgl[][][][])
                      }
                      frame 3 {
                        n884 = Unbundle By Name(w766) -> ("D Img Focus Index"=w765:sgl[][])
                        n885 = Unbundle By Name(w764) -> ("D Img Focus Index array"=w763:sgl[][][][])
                      }
                    }
                    n886 = local write "Status message"("Single scan finished." ("Status message")) -> ()
                    n887 = local write "Focus Index tiled"(w745) -> ()
                    n888 = local write "Focus Index array tiled"(w744) -> ()
                    n889 = local write "Scan x1"(FALSE ("Scan")) -> ()
                  }
                }
              }
            }
          }
        }
        n890 = local read "Stop"() -> (w717:bool)
      }
      n891 = while {
        stop <- w5425 stop-if-true
        n892 = stacked-sequence {
          tunnel: [_ w5452] -> w5425
          frame #0 {
            n893 = local read "Unfreeze"() -> (w5427:bool)
            n894 = case shown="True" w5427 {
              frame False {
              }
              frame True {
                n895 = stacked-sequence {
                  frame #0 {
                    w5429 = T44."Disabled and Grayed Out" ("Disabled")
                    n896 = local read "FIB HW Config"() -> (w5435:T23)
                    n897 = local read "FIB HW Config"() -> (w5432:T23)
                    n898 = local read "Api"() -> (w5428:refnum<k7>)
                    n899 = Unbundle By Name(w5435) -> ("Beam blank"=w5434:tag)
                    n900 = Unbundle By Name(w5432) -> ("FIB Ext Scan"=w5430:tag)
                    n901 = call "FIB beam blank.vi"("Api"=w5428, "Beam blanked"=TRUE, "lines"=w5434) -> ()  [unwired: 2 in, 1 out]
                    n902 = call "FIB ext scan.vi"("Ext on"=TRUE ("data"), "FIB Ext Scan"=w5430) -> ()  [unwired: 9 in, 1 out]
                    n903 = property on="Pre image" class="Bool (strict)"("DisabledEnum"=w5429) -> ()  [unwired: 2 in, 2 out]
                    n904 = property on="Post image" class="Bool (strict)"("DisabledEnum"=w5429) -> ()  [unwired: 2 in, 2 out]
                  }
                  frame #1 {
                    n905 = local read "COM port"() -> (w5437:refnum<visa-resource-name>)
                    n906 = local read "FIB HW Config"() -> (w5438:T23)
                    n907 = local read "FIB Options"() -> (w5441:T33)
                    n908 = local read "FIB single scan"() -> (w5436:bool)
                    n909 = local read "FIB Scan Parameters"() -> (w5442:T32)
                    n910 = call "FIB realtime imaging PXIe-6124.vi"("HW Config"=w5438, "Options"=w5441, "Single scan"=w5436, "Scan Para"=w5442, "As subVi"=TRUE, "COM port"=w5437) -> ("error out"=w5440:errorcluster)  [unwired: 3 in, 1 out]
                    n911 = Unbundle By Name(w5441) -> ("Scan mode"=w5443:u16)
                    n912 = Unbundle By Name(w5442) -> ("X resolution"=w5445:u32, "Z resolution"=w5444:u32)
                    n913 = Unbundle By Name(w5440) -> ("status"=w5439:bool)
                    n914 = Equal To 0?(x=w5443) -> (x = 0?=w5447:bool)
                    n915 = Bundle("X resolution"=w5445, "Z resolution"=w5444) -> (w5446:cluster{"X resolution":u32, "Z resolution":u32})  [unwired: 1 in]
                    n916 = property on="X resolution with rampdown" class="DigNum (strict)"("Visible"=w5447) -> ()  [unwired: 2 in, 2 out]
                    n917 = case shown="True" w5439 {
                      frame False {
                      }
                      frame True {
                        n918 = local write "Unfreeze"(FALSE ("Freeze")) -> ()
                      }
                    }
                    n919 = property on="FIB Image" class="IntGraph (strict)"("Plot Area Size"=w5446) -> ()  [unwired: 2 in, 2 out]
                  }
                  frame #2 {
                    n920 = local read "FIB single scan"() -> (w5450:bool)
                    n921 = case shown="True" w5450 {
                      frame False {
                      }
                      frame True {
                        w5451 = FALSE ("FIB single scan")
                        n922 = local write "FIB single scan"(w5451) -> ()
                        n923 = local write "FIB Imaging"(w5451) -> ()
                        n924 = local write "Unfreeze"(w5451) -> ()
                      }
                    }
                  }
                }
              }
            }
          }
          frame #1 {
            n925 = local read "Stop"() -> (w5452:bool)
            n926 = case shown="True" w5452 {
              frame False {
              }
              frame True {
                n927 = local read "FIB HW Config"() -> (w5456:T23)
                n928 = Unbundle By Name(w5456) -> ("Beam blank"=w5455:tag)
                n929 = local read "Api"() -> (w5453:refnum<k7>)
                n930 = call "FIB beam blank.vi"("Api"=w5453, "Beam blanked"=TRUE, "lines"=w5455) -> ()  [unwired: 2 in, 1 out]
              }
            }
          }
        }
        n931 = Wait Until Next ms Multiple(millisecond multiple=u32 100) -> ()  [unwired: 1 out]
      }
      n932 = while {
        stop <- w5458 stop-if-true
        n933 = case shown="True" "FIB" {
          tunnel: [w5470 w5478] -> w5458
          frame False {
            w5462 = u8 0 ("AF Count")
            w5465 = sgl[][][] [] ("FI grid array")
            w5466 = FALSE ("Rect Milling Line Paused")
            w5460 = T44."Enabled" ("Disabled")
            n934 = local write "AF Count"(w5462) -> ()
            n935 = local write "AS Count"(w5462) -> ()
            n936 = local write "AA Count"(w5462) -> ()
            n937 = local write "Skip Steps tiled"(u8[][] [] ("Skip Steps tiled")) -> ()
            n938 = local write "Stig Options"(enum16{"Defaut", "Stig X", "Stig Y"}."Defaut" ("Stig Options")) -> ()
            n939 = local write "Auto Focus"(w5466) -> ()
            n940 = local write "Auto Stig"(w5466) -> ()
            n941 = local write "Auto Align"(w5466) -> ()
            n942 = local write "Mill Manual Pause"(w5466) -> ()
            n943 = local write "Mill Stop"(w5466) -> ()
            n944 = local write "Pause for reheat"(w5466) -> ()
            n945 = local read "Stop"() -> (w5470:bool)
            n946 = local write "FI grid array"(w5465) -> ()
            n947 = local write "FI array tiled"(w5465) -> ()
            n948 = local write "WD array tiled"(w5465) -> ()
            n949 = local write "StigX array tiled"(w5465) -> ()
            n950 = local write "StigY array tiled"(w5465) -> ()
            n951 = local write "AlnX array tiled"(w5465) -> ()
            n952 = local write "AlnY array tiled"(w5465) -> ()
            n953 = shared-variable "My Computer\\Zeiss Library.lvlib\\Milling Stop"(w5470) -> ()  [unwired: 1 in, 1 out]
            n954 = local write "Aln Options"(enum16{"Defaut", "Aln X", "Aln Y"}."Defaut" ("Aln Options")) -> ()
            n955 = property on="Mill start from Last" class="Bool (strict)"("DisabledEnum"=w5460) -> ()  [unwired: 2 in, 2 out]
            n956 = property on="Keep aspect ratio" class="Bool (strict)"("DisabledEnum"=w5460) -> ()  [unwired: 2 in, 2 out]
            n957 = property on="X Grids" class="Arr (strict)"("DisabledEnum"=w5460) -> ()  [unwired: 2 in, 2 out]
            n958 = property on="Y Grids" class="Arr (strict)"("DisabledEnum"=w5460) -> ()  [unwired: 2 in, 2 out]
            n959 = property on="Primary X index" class="Arr (strict)"("DisabledEnum"=w5460) -> ()  [unwired: 2 in, 2 out]
            n960 = property on="Primary Y index" class="Arr (strict)"("DisabledEnum"=w5460) -> ()  [unwired: 2 in, 2 out]
            n961 = property on="Scan x1" class="Bool (strict)"("DisabledEnum"=w5460) -> ()  [unwired: 2 in, 2 out]
            n962 = property on="Scan xn" class="Bool (strict)"("DisabledEnum"=w5460) -> ()  [unwired: 2 in, 2 out]
            n963 = property on="FIB Imaging" class="Bool (strict)"("DisabledEnum"=w5460) -> ()  [unwired: 2 in, 2 out]
            n964 = property on="FIB time lapse" class="Bool (strict)"("DisabledEnum"=w5460) -> ()  [unwired: 2 in, 2 out]
            n965 = property on="Auto Focus" class="Bool (strict)"("DisabledEnum"=w5460) -> ()  [unwired: 2 in, 2 out]
            n966 = property on="Auto Stig" class="Bool (strict)"("DisabledEnum"=w5460) -> ()  [unwired: 2 in, 2 out]
            n967 = property on="Auto Align" class="Bool (strict)"("DisabledEnum"=w5460) -> ()  [unwired: 2 in, 2 out]
            n968 = property on="Reset" class="Bool (strict)"("DisabledEnum"=w5460) -> ()  [unwired: 2 in, 2 out]
